vi "DropIn Get Button Clicks - Solution.vi"(0 "VI Refnum":refnum<vi>, 5 "file path":path=path "C:/Solutions/Advanced Architectures in LabVIEW/Test Drop In.txt", 11 "error in (no error)":errorcluster) -> (15 "error out":errorcluster)   [LabVIEW 2011]
doc: "This is the solution to the exercise.\n\nAAL 9/09"
uses:
  <vilib>/Utility/traverseref.llb/TRef TravTarget.ctl
  <vilib>/Utility/traverseref.llb/VI Scripting - Traverse.lvlib
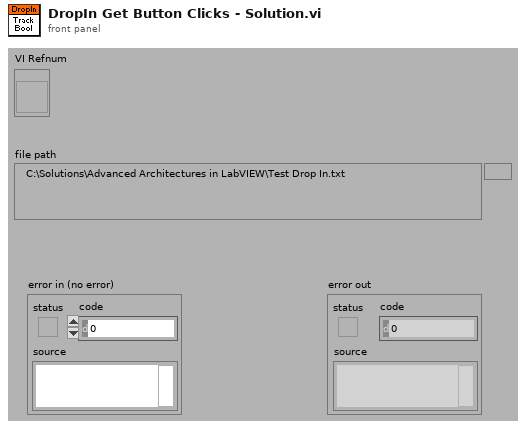
[diagram p1: front panel]
types:
  T1 = typedef "TRef TravTarget.ctl" = enum16{"FP", "BD", "Other"}
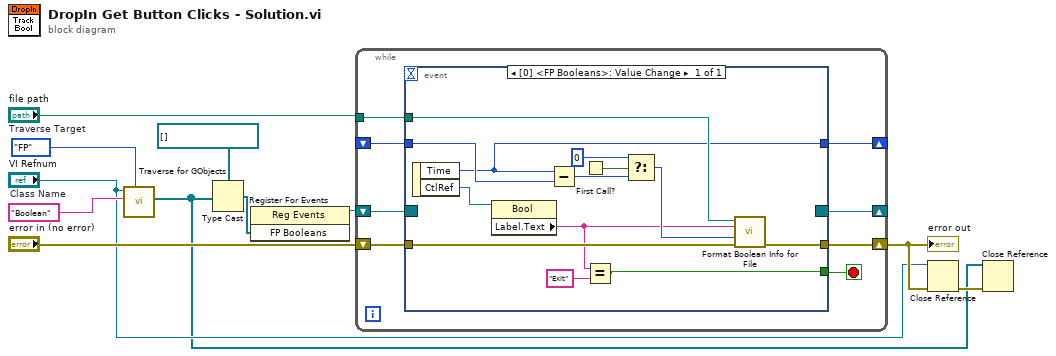
[diagram p0: block diagram]
diagram:
  w6 = "Boolean"  # Class Name
  w7 = TRef_TravTarget."FP"  # Traverse Target
  n1 = call <vilib>:"Traverse for GObjects.vi"("Traverse Target"=w7, "Class Name"=w6, "VI Refnum"="VI Refnum") -> ("References"=w1:refnum<vi>[])  [unwired: 5 in, 3 out]
  n2 = Type Cast(type=refnum<vi>[] [] ("FP Booleans"), x=w1) -> (*(type *) &x=w3:refnum<vi>[])
  n3 = register-events(w3) -> (reference out=w4:refnum<event-registration>)  [unwired: 2 in, 1 out]
  n4 = while {
    shift-right: [w16] -> _
    shift-left: w4 -> [w19]
    shift-right: [w17] -> w10
    shift-left: "error in (no error)" -> [w18]
    tunnel: "file path" -> [w15]
    shift-right: [w13] -> _
    shift-left: _ -> [w14]
    stop <- w12 stop-if-true
    n5 = event shown="[0] <FP Booleans>: Value Change" {
      selector: w19 -> [_]
      dyn-events: [_] -> w16
      timeout: _ -> [_]
      tunnel: w18 -> [w31]
      tunnel: [w30] -> w17
      tunnel: w15 -> [w29]
      tunnel: w14 -> [w32]
      tunnel: [w28] -> w13
      tunnel: [w20] -> w12
      event Value Change {
        n6 = event-data() -> ("Time"=w28:u32, "CtlRef"=w23:refnum<vi>)  [unwired: 1 out]
        n7 = property class="Bool"(reference=w23) -> ("Label.Text"=w22:string)  [unwired: 1 in, 2 out]
        n8 = Subtract(x=w28, y=w32) -> (x-y=w26:u32)
        n9 = First Call?() -> (First Call?: T/F=w27:bool)
        n10 = Equal?(x=w22, y="Exit") -> (x = y?=w20:bool)
        n11 = Select(t=u32 0, s=w27, f=w26) -> (s? t:f=w25:u32)
        n12 = call "Format Boolean Info for File.vi"("File Name"=w29, "Label Name"=w22, "Time (msec)"=w25, "error in (no error)"=w31) -> ("error out"=w30:errorcluster)  [unwired: 1 in, 5 out]
      }
    }
  }
  "error out" <- w10
  n13 = Close Reference(reference="VI Refnum", error in (no error)=w10) -> (error out=w9:errorcluster)
  n14 = Close Reference(reference=w1, error in (no error)=w9) -> ()  [unwired: 1 out]
